vi "Read Message.vi"(8 "error in (no error)":errorcluster, 11 "Muon Detector in":refnum<class "Muon Detector.lvclass">) -> (0 "error out":errorcluster, 2 "Message":string, 3 "Muon Detector out":refnum<class "Muon Detector.lvclass">)   [LabVIEW 2019, in "Muon Detector.lvclass"]
uses:
  Muon Detector.lvclass
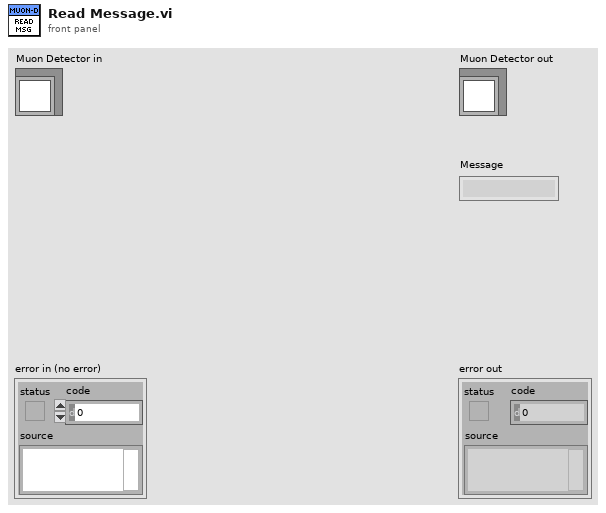
[diagram p1: front panel]
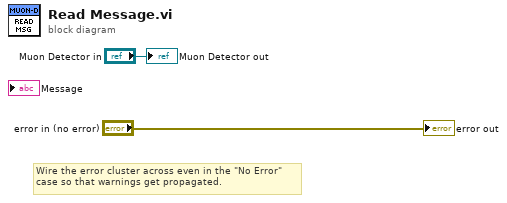
[diagram p0: block diagram]
diagram:
  # "Wire the error cluster across even in the \"No Error\"\ncase so that warnings get propagated."
  "error out" <- "error in (no error)"
  "Muon Detector out" <- "Muon Detector in"
